vi "Controller_ChannelLookup_Test.vi"() -> ()   [LabVIEW 2010]
uses:
  labbCAN_Bus_API/labbCAN_Bus_API.lvlib
  labbCAN_Controller_API/labbCAN_Controller_API.lvlib
panel:
  out "Controller Channels":string[](array[string])
  out "Control Channel Count":i32
  out "error out":errorcluster caption="Fehler (Ausgang)"
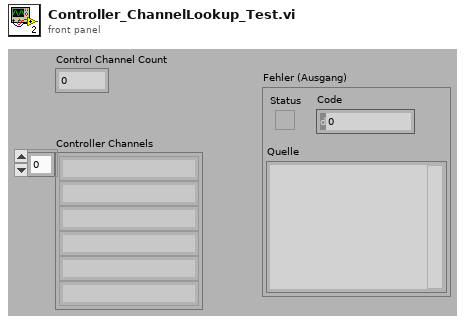
[diagram p1: front panel]
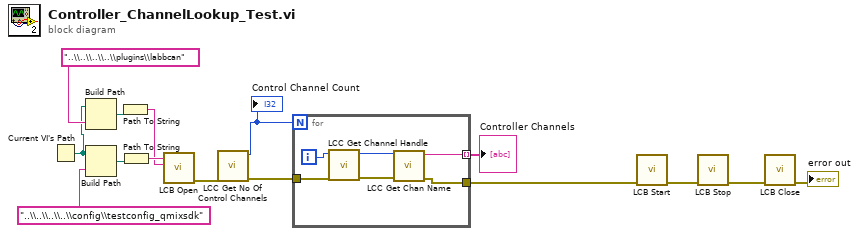
[diagram p0: block diagram]
diagram:
  n1 = Current VI's Path() -> (path=w6:path)
  n2 = Build Path(base path=w6, name or relative path="..\\..\\..\\..\\plugins\\labbcan" ("Name oder relativer Pfad")) -> (appended path=w8:path)
  n3 = Build Path(base path=w6, name or relative path="..\\..\\..\\..\\config\\testconfig_qmixsdk" ("Name oder relativer Pfad")) -> (appended path=w11:path)
  n4 = Path To String(path=w8) -> (string=w5:string)
  n5 = Path To String(path=w11) -> (string=w14:string)
  n6 = call "LCB Open.vi"("PluginSearchPath"=w5, "Device Configuration Path"=w14) -> ("error out"=w9:errorcluster)  [unwired: 9 in]
  n7 = call "LCC Get No Of Control Channels.vi"("error in (no error)"=w9) -> ("error out"=w3:errorcluster, "Control Channel Count"=w4:i32)  [unwired: 9 in]
  "Control Channel Count" <- w4
  n8 = for {
    N: w4 -> [_]
    tunnel: w3 -> [w18]
    tunnel: [w17] -> w2
    tunnel: [w16] -> w1 mode=indexing
    i -> [w19]
    n9 = call "LCC Get Channel Handle.vi"("error in (no error)"=w18, "Index"=w19) -> ("error out"=w21:errorcluster, "Control Channel"=w20:i64)  [unwired: 8 in]
    n10 = call "LCC Get Chan Name.vi"("error in (no error)"=w21, "Channel Handle"=w20) -> ("error out"=w17:errorcluster, "Channel Name"=w16:string)  [unwired: 8 in]
  }
  "Controller Channels" <- w1
  n11 = call "LCB Start.vi"("error in (no error)"=w2) -> ("error out"=w10:errorcluster)  [unwired: 10 in]
  n12 = call "LCB Stop.vi"("error in (no error)"=w10) -> ("error out"=w13:errorcluster)  [unwired: 10 in]
  n13 = call "LCB Close.vi"("error in (no error)"=w13) -> ("error out"=→"error out":errorcluster)  [unwired: 10 in]
